vi "UI_(04A)_Set_Stop_State.vi"(3 "error in (no error)":errorcluster, 4 "Settings cluster in":T1={"Defaults"={"Default User"=0.0, "VISA Resource Name "=""}, "Recording and saving"={"Researcher name"="", "Name prefix"="", "Data post-processing"={"Filter type"=enum."Savitzky-Golay", "Length"=31, "Order"=3}, "Stop at"=0.0, "\"Stop at\" enabled"=FALSE, "Default save folder path"=path "", "Acquisition FPS"=enum."Max"}, "Geometry"={"Cage diameter, mm"=0, "Starting angle MIDFIELD"=0, "Starting angle BORDER"=0, "Radius, mm CENTER"=0, "Radius, mm MIDFIELD"=0, "N segments MIDFIELD"=0, "N segments BORDER"=0, "R-gap, mm"=0.0, "Bridge swap"=FALSE, "Bridge H. offset"=0.0, "Bridge V. offset"=0.0, "Twisted neck"=FALSE, "Alt. magn. orientation"=FALSE, "Sensor board size"=enum."Small"}, "IO parameters"={"IO general config."=0, "IO 1 configuration"=0, "IO 2 configuration"=0, "IO 3 configuration"=0, "IO 4 configuration"=0, "Activate ext. RS-232"=0, "IO inversion config."=0, "Sync capability"=1}, "Conditions presets array"=[{"Enabled"=FALSE, "Name"="", "Specifier(s)"=[], "Response"={"Response type"=enum."None", "TTL pulse length, ms"=0.0}}, {"Enabled"=FALSE, "Name"="", "Specifier(s)"=[], "Response"={"Response type"=enum."None", "TTL pulse length, ms"=0.0}}, {"Enabled"=FALSE, "Name"="", "Specifier(s)"=[], "Response"={"Response type"=enum."None", "TTL pulse length, ms"=0.0}}, {"Enabled"=FALSE, "Name"="", "Specifier(s)"=[], "Response"={"Response type"=enum."None", "TTL pulse length, ms"=0.0}}, {"Enabled"=FALSE, "Name"="", "Specifier(s)"=[], "Response"={"Response type"=enum."None", "TTL pulse length, ms"=0.0}}, {"Enabled"=FALSE, "Name"="", "Specifier(s)"=[], "Response"={"Response type"=enum."None", "TTL pulse length, ms"=0.0}}, {"Enabled"=FALSE, "Name"="", "Specifier(s)"=[], "Response"={"Response type"=enum."None", "TTL pulse length, ms"=0.0}}, {"Enabled"=FALSE, "Name"="", "Specifier(s)"=[], "Response"={"Response type"=enum."None", "TTL pulse length, ms"=0.0}}, {"Enabled"=FALSE, "Name"="", "Specifier(s)"=[], "Response"={"Response type"=enum."None", "TTL pulse length, ms"=0.0}}, {"Enabled"=FALSE, "Name"="", "Specifier(s)"=[], "Response"={"Response type"=enum."None", "TTL pulse length, ms"=0.0}}, {"Enabled"=FALSE, "Name"="", "Specifier(s)"=[], "Response"={"Response type"=enum."None", "TTL pulse length, ms"=0.0}}, {"Enabled"=FALSE, "Name"="", "Specifier(s)"=[], "Response"={"Response type"=enum."None", "TTL pulse length, ms"=0.0}}, {"Enabled"=FALSE, "Name"="", "Specifier(s)"=[], "Response"={"Response type"=enum."None", "TTL pulse length, ms"=0.0}}, {"Enabled"=FALSE, "Name"="", "Specifier(s)"=[], "Response"={"Response type"=enum."None", "TTL pulse length, ms"=0.0}}], "Calibration parameters"={"Timing calibration sw/hw"=1.0, "True FPS"=80.0, "True frame time, s"=80.0, "Disp. calibration info"=[]}, "Settings loaded OK"=FALSE} {"Calibration parameters"."True frame time, s" format="%.10g"; "Calibration parameters"."Disp. calibration info"."Speed, µl per ms" format="%.3g"; "Calibration parameters"."True FPS" format="%.10g"; "Calibration parameters"."Timing calibration sw/hw" format="%.10g"; "Conditions presets array"."Response"."TTL pulse length, ms" min=0.0 max=10000.0 step=10.0 format="%0.0g"; "Conditions presets array"."Specifier(s)"."Validity criteria(s)"."Validity value" min=0.0 step=0.1 format="%.2g"; "Conditions presets array"."Specifier(s)"."Value" step=1.0 format="%#.2g"; "Recording and saving"."Data post-processing"."Order" min=3 max=11 step=2; "Recording and saving"."Data post-processing"."Length" min=5 max=301 step=2; "Geometry"."Cage diameter, mm" scale=0.0..340.0}, 5 "All references in":T16) -> (0 "error out":errorcluster, 1 "Settings cluster out":T1={"Defaults"={"Default User"=0.0, "VISA Resource Name "=""}, "Recording and saving"={"Researcher name"="", "Name prefix"="", "Data post-processing"={"Filter type"=enum."Savitzky-Golay", "Length"=31, "Order"=3}, "Stop at"=0.0, "\"Stop at\" enabled"=FALSE, "Default save folder path"=path "", "Acquisition FPS"=enum."Max"}, "Geometry"={"Cage diameter, mm"=0, "Starting angle MIDFIELD"=0, "Starting angle BORDER"=0, "Radius, mm CENTER"=0, "Radius, mm MIDFIELD"=0, "N segments MIDFIELD"=0, "N segments BORDER"=0, "R-gap, mm"=0.0, "Bridge swap"=FALSE, "Bridge H. offset"=0.0, "Bridge V. offset"=0.0, "Twisted neck"=FALSE, "Alt. magn. orientation"=FALSE, "Sensor board size"=enum."Small"}, "IO parameters"={"IO general config."=0, "IO 1 configuration"=0, "IO 2 configuration"=0, "IO 3 configuration"=0, "IO 4 configuration"=0, "Activate ext. RS-232"=0, "IO inversion config."=0, "Sync capability"=1}, "Conditions presets array"=[{"Enabled"=FALSE, "Name"="", "Specifier(s)"=[], "Response"={"Response type"=enum."None", "TTL pulse length, ms"=0.0}}, {"Enabled"=FALSE, "Name"="", "Specifier(s)"=[], "Response"={"Response type"=enum."None", "TTL pulse length, ms"=0.0}}, {"Enabled"=FALSE, "Name"="", "Specifier(s)"=[], "Response"={"Response type"=enum."None", "TTL pulse length, ms"=0.0}}, {"Enabled"=FALSE, "Name"="", "Specifier(s)"=[], "Response"={"Response type"=enum."None", "TTL pulse length, ms"=0.0}}, {"Enabled"=FALSE, "Name"="", "Specifier(s)"=[], "Response"={"Response type"=enum."None", "TTL pulse length, ms"=0.0}}, {"Enabled"=FALSE, "Name"="", "Specifier(s)"=[], "Response"={"Response type"=enum."None", "TTL pulse length, ms"=0.0}}, {"Enabled"=FALSE, "Name"="", "Specifier(s)"=[], "Response"={"Response type"=enum."None", "TTL pulse length, ms"=0.0}}, {"Enabled"=FALSE, "Name"="", "Specifier(s)"=[], "Response"={"Response type"=enum."None", "TTL pulse length, ms"=0.0}}, {"Enabled"=FALSE, "Name"="", "Specifier(s)"=[], "Response"={"Response type"=enum."None", "TTL pulse length, ms"=0.0}}, {"Enabled"=FALSE, "Name"="", "Specifier(s)"=[], "Response"={"Response type"=enum."None", "TTL pulse length, ms"=0.0}}, {"Enabled"=FALSE, "Name"="", "Specifier(s)"=[], "Response"={"Response type"=enum."None", "TTL pulse length, ms"=0.0}}, {"Enabled"=FALSE, "Name"="", "Specifier(s)"=[], "Response"={"Response type"=enum."None", "TTL pulse length, ms"=0.0}}, {"Enabled"=FALSE, "Name"="", "Specifier(s)"=[], "Response"={"Response type"=enum."None", "TTL pulse length, ms"=0.0}}, {"Enabled"=FALSE, "Name"="", "Specifier(s)"=[], "Response"={"Response type"=enum."None", "TTL pulse length, ms"=0.0}}], "Calibration parameters"={"Timing calibration sw/hw"=1.0, "True FPS"=80.0, "True frame time, s"=80.0, "Disp. calibration info"=[]}, "Settings loaded OK"=FALSE} {"Calibration parameters"."True frame time, s" format="%.10g"; "Calibration parameters"."Disp. calibration info"."Speed, µl per ms" format="%.3g"; "Calibration parameters"."True FPS" format="%.10g"; "Calibration parameters"."Timing calibration sw/hw" format="%.10g"; "Conditions presets array"."Response"."TTL pulse length, ms" min=0.0 max=10000.0 step=10.0 format="%0.0g"; "Conditions presets array"."Specifier(s)"."Validity criteria(s)"."Validity value" min=0.0 step=0.1 format="%.2g"; "Conditions presets array"."Specifier(s)"."Value" step=1.0 format="%#.2g"; "Recording and saving"."Data post-processing"."Order" min=3 max=11 step=2; "Recording and saving"."Data post-processing"."Length" min=5 max=301 step=2; "Geometry"."Cage diameter, mm" scale=0.0..340.0}, 2 "All references out":T16)   [LabVIEW 2018, in "Tracker.lvlib"]
uses:
  Tracker.lvlib
  Controls/CTL_All_References.ctl
  Controls/CTL_Controls_References.ctl
  Controls/CTL_Indicators_References.ctl
  Controls/CTL_Panes_and_VIs_References.ctl
  Controls/CTL_Histogram_Properties.ctl
  <vilib>/Utility/miscctls.llb/LVRangeTypeDef.ctl
  Controls/CTL_Settings_cluster.ctl
  Controls/CTL_Filter_selector.ctl
  Controls/CTL_Acquisition_speed_selector.ctl
  Controls/CTL_Segmented_plot_parameters.ctl
  Controls/CTL_IO_params_cluster.ctl
  Controls/CTL_Conditions_Array.ctl
  Controls/CTL_Conditions_Cluster.ctl
  Controls/CTL_Condition_type.ctl
  Controls/CTL_Comparison_type.ctl
  Controls/CTL_Validity_check_criteria.ctl
  Controls/CTL_Condition_response_type.ctl
  Controls/CTL_Calibration_parameters.ctl
  Controls/CTL_Dispenser_calibration_info.ctl
  <vilib>/Utility/error.llb/Error Cluster From Error Code.vi
  <vilib>/ErrorRing/Error Ring.xnode
panel:
  in  "Histogram initialization cluster":T14={"X Scale.Range"={"Minimum"=0.0, "Maximum"=13.0, "Increment"=1.0, "Minor Increment"=1.0, "Start"=0.0}, "Caption.Text"="Zone preference (normalized)", "X Scale.Offset and Multiplier:Multiplier"=1.0, "X Scale.Offset and Multiplier:Offset"=0.0, "X Scale.Scale Fit"=2, "X Scale.Display Format:Precision"=0, "Y Scale.Mapping Mode"=0, "Zones preference empty initialized array"=[0, 0, 0, 0, 0, 0, 0, 0, 0, 0, 0, 0, 0, 0], "Plot.Fill/Point Color"=15790320}
  out "Panes references":T19
  out "Controls references params":string[][](array[string])
  out "Indicators references params":string[][](array[string])
  out "Indicators references":T18
  out "Controls references":T17
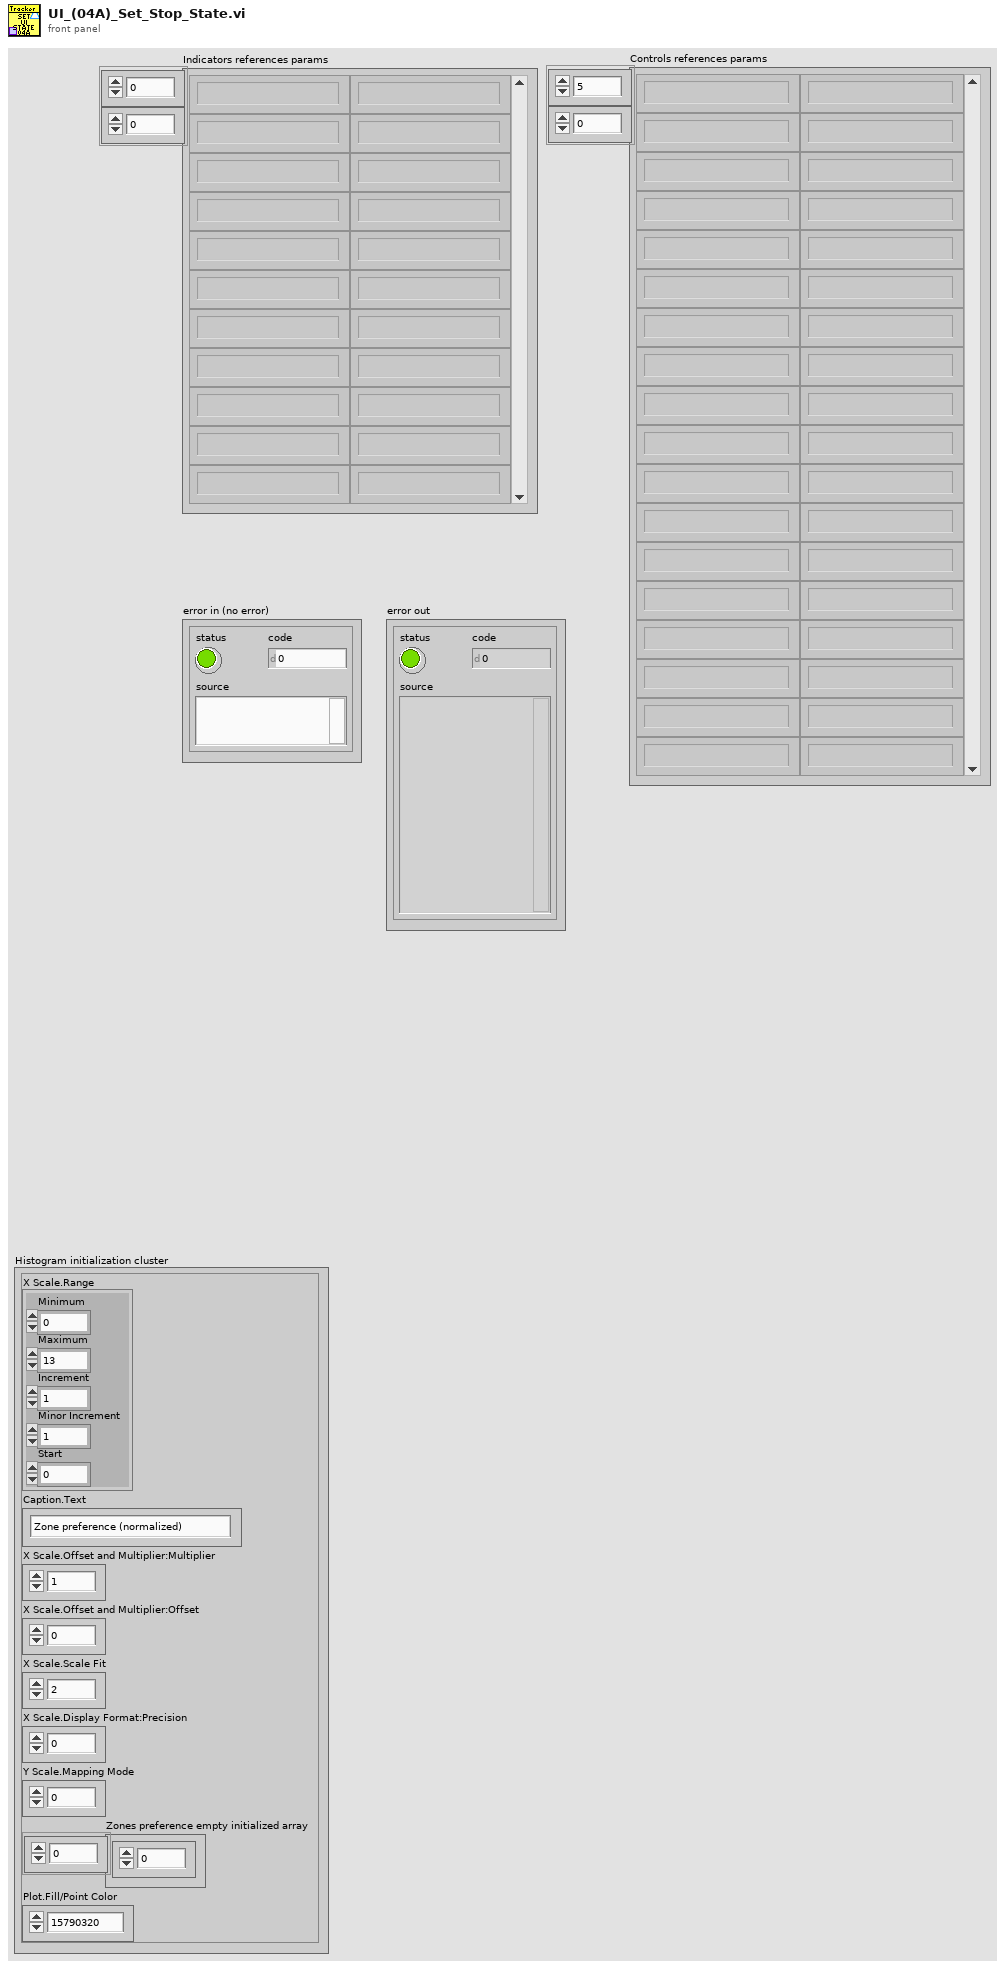
[diagram p1: front panel]
types:
  T1 = typedef "Tracker.lvlib/CTL_Settings_cluster.ctl" = cluster{"Defaults":cluster{"Default User":dbl, "VISA Resource Name ":string}, "Recording and saving":cluster{"Researcher name":string, "Name prefix":string, "Data post-processing":T2, "Stop at":dbl, "\"Stop at\" enabled":bool, "Default save folder path":path, "Acquisition FPS":T3}, "Geometry":T4, "IO parameters":T5, "Conditions presets array":T6, "Calibration parameters":T12, "Settings loaded OK":bool}
  T2 = typedef "Tracker.lvlib/CTL_Filter_selector.ctl" = cluster{"Filter type":enum16{"None", "Savitzky-Golay"}, "Length":i32, "Order":i32}
  T3 = typedef "Tracker.lvlib/CTL_Acquisition_speed_selector.ctl" = enum16{"Max", "Optimal", "Eco"}
  T4 = typedef "Tracker.lvlib/CTL_Segmented_plot_parameters.ctl" = cluster{"Cage diameter, mm":u16, "Starting angle MIDFIELD":i16, "Starting angle BORDER":i16, "Radius, mm CENTER":u16, "Radius, mm MIDFIELD":u16, "N segments MIDFIELD":u8, "N segments BORDER":u8, "R-gap, mm":sgl, "Bridge swap":bool, "Bridge H. offset":sgl, "Bridge V. offset":sgl, "Twisted neck":bool, "Alt. magn. orientation":bool, "Sensor board size":enum16{"Small", "Large"}}
  T5 = typedef "Tracker.lvlib/CTL_IO_params_cluster.ctl" = cluster{"IO general config.":u16, "IO 1 configuration":u16, "IO 2 configuration":u16, "IO 3 configuration":u16, "IO 4 configuration":u16, "Activate ext. RS-232":u16, "IO inversion config.":u16, "Sync capability":u8}
  T6 = typedef "Tracker.lvlib/CTL_Conditions_Array.ctl" = T7[]
  T7 = typedef "Tracker.lvlib/CTL_Conditions_Cluster.ctl" = cluster{"Enabled":bool, "Name":string, "Specifier(s)":cluster{"Specifier enabled":bool, "Condition type":T8, "Limit type":T9, "Value":dbl, "Validity criteria(s)":cluster{"V. check enabled":bool, "Criteria":T10, "Validity value":dbl}[]}[], "Response":cluster{"Response type":T11, "TTL pulse length, ms":dbl}}
  T8 = typedef "Tracker.lvlib/CTL_Condition_type.ctl" = enum16{"Not in use", "Speed", "Zone", "Angle to wall"}
  T9 = typedef "Tracker.lvlib/CTL_Comparison_type.ctl" = enum16{"Less", "Less or Equal", "Equal", "Greater or Equal", "Greater", "Not Equal"}
  T10 = typedef "Tracker.lvlib/CTL_Validity_check_criteria.ctl" = enum16{"Running bout (seconds)", "Running bout (meters)"}
  T11 = typedef "Tracker.lvlib/CTL_Condition_response_type.ctl" = enum16{"None", "TTL"}
  T12 = typedef "Tracker.lvlib/CTL_Calibration_parameters.ctl" = cluster{"Timing calibration sw/hw":dbl, "True FPS":dbl, "True frame time, s":dbl, "Disp. calibration info":T13}
  T13 = typedef "Tracker.lvlib/CTL_Dispenser_calibration_info.ctl" = cluster{"Channel":u8, "Speed, µl per ms":dbl}[]
  T14 = typedef "Tracker.lvlib/CTL_Histogram_Properties.ctl" = cluster{"X Scale.Range":T15, "Caption.Text":string, "X Scale.Offset and Multiplier:Multiplier":dbl, "X Scale.Offset and Multiplier:Offset":dbl, "X Scale.Scale Fit":u8, "X Scale.Display Format:Precision":u8, "Y Scale.Mapping Mode":u8, "Zones preference empty initialized array":i32[], "Plot.Fill/Point Color":u32}
  T15 = typedef "LVRangeTypeDef.ctl" = cluster{"Minimum":dbl, "Maximum":dbl, "Increment":dbl, "Minor Increment":dbl, "Start":dbl}
  T16 = typedef "Tracker.lvlib/CTL_All_References.ctl" = cluster{"Controls references":T17, "Indicators references":T18, "Service references":T19}
  T17 = typedef "Tracker.lvlib/CTL_Controls_References.ctl" = cluster{"Check HW connection":refnum<vi>, "Save settings":refnum<vi>, "Reset zones":refnum<vi>, "Reset stimuli":refnum<vi>, "Record/Stop":refnum<vi>, "Reset barplot":refnum<vi>, "Multiplyer of chart RX":refnum<vi>, "Show zones":refnum<vi>, "Show magnets":refnum<vi>, "Show heatmap":refnum<vi>, "Show full track":refnum<vi>, "Open File":refnum<vi>, "Play/Pause":refnum<vi>, "Trace, s":refnum<vi>, "Playback speed":refnum<vi>, "Timeline":refnum<vi>, "By Zone stim. setup":refnum<vi>, "Set/Rec and Analyse Tab":refnum<vi>, "Cage radial segmentation":refnum<vi>, "Set IO config":refnum<vi>, "Rainbow (time)":refnum<vi>, "Rainbow (speed)":refnum<vi>, "Add Reward":refnum<vi>, "Modify Reward":refnum<vi>, "Delete Reward":refnum<vi>}
  T18 = typedef "Tracker.lvlib/CTL_Indicators_References.ctl" = cluster{"HW info":refnum<vi>, "Port":refnum<vi>, "Ready":refnum<vi>, "IO status indicator":refnum<vi>, "Current Time":refnum<vi>, "Record timestamp":refnum<vi>, "Mouse speed":refnum<vi>, "Mouse speed, mm/s":refnum<vi>, "Running, perc. of time":refnum<vi>, "Histograms":refnum<vi>, "Cage size":refnum<vi>, "Reward":refnum<vi>}
  T19 = typedef "Tracker.lvlib/CTL_Panes_and_VIs_References.ctl" = cluster{"Pane":refnum<vi>, "This VI":refnum<vi>, "Menu":refnum<k9>}
  T20 = enum8{"Enabled", "Disabled", "Disabled and Grayed Out"}
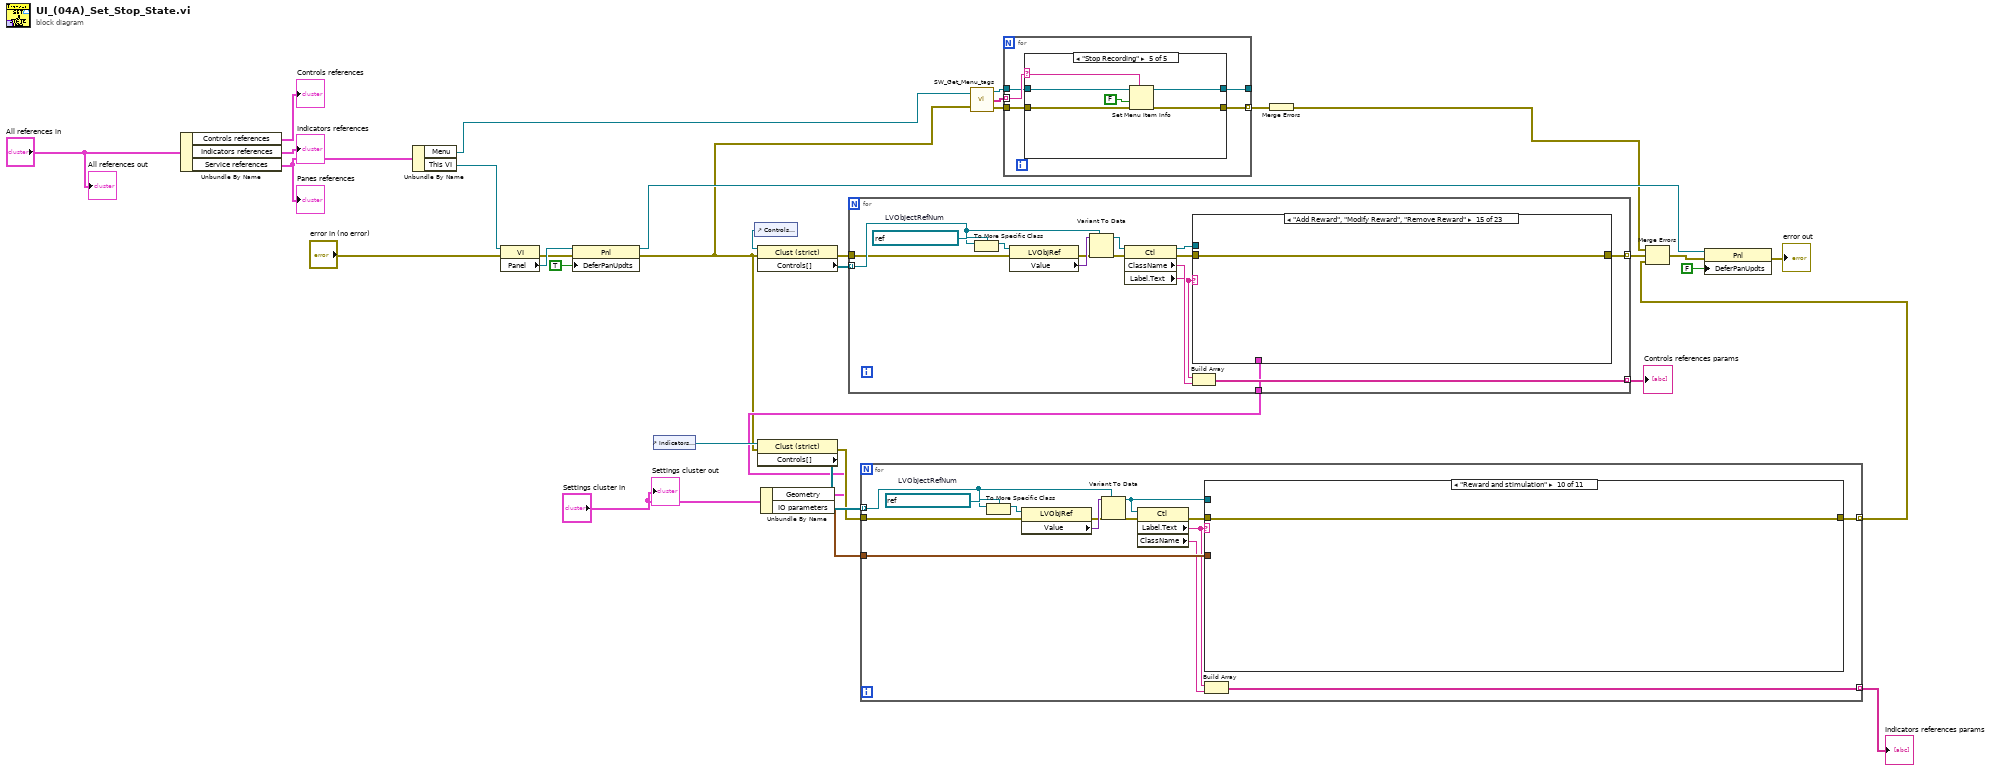
[diagram p0: block diagram]
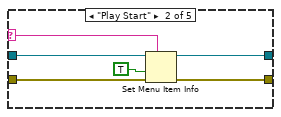
[diagram p3: hidden frame]
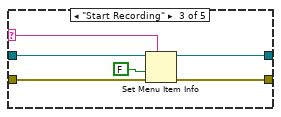
[diagram p4: hidden frame]
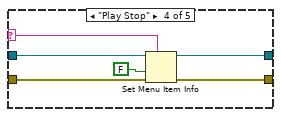
[diagram p5: hidden frame]
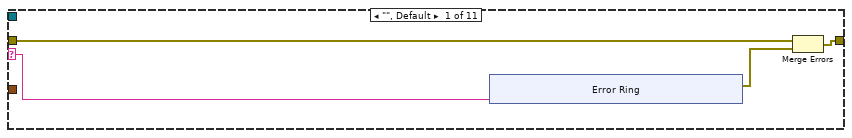
[diagram p6: hidden frame]
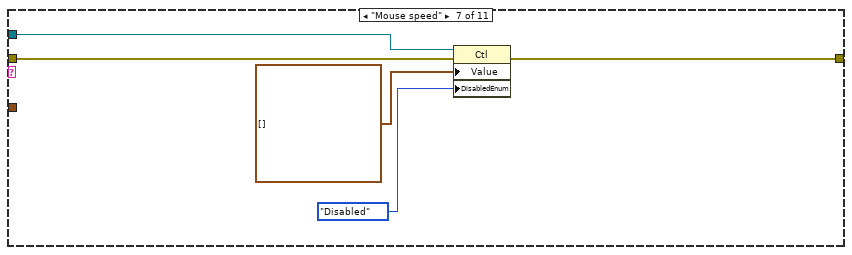
[diagram p12: hidden frame]
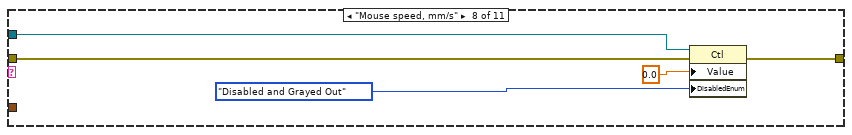
[diagram p13: hidden frame]
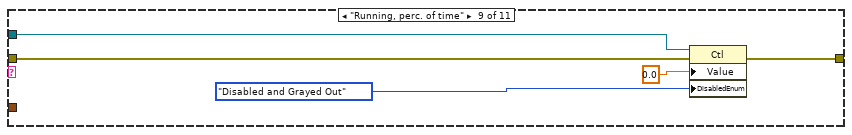
[diagram p14: hidden frame]
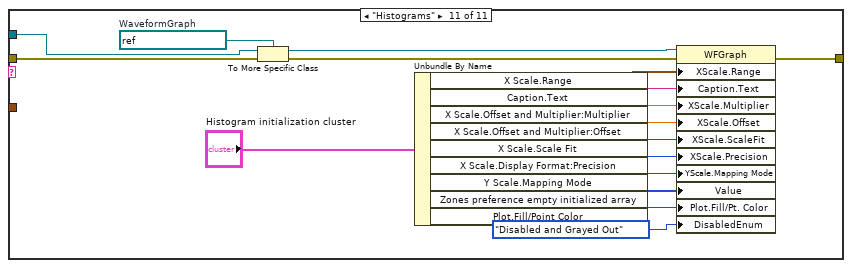
[diagram p15: hidden frame]
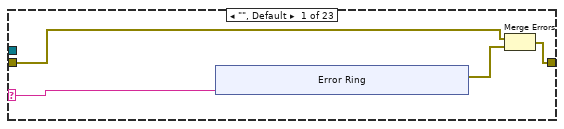
[diagram p16: hidden frame]
diagram:
  n1 = Unbundle By Name("All references in") -> ("Controls references"=→"Controls references":T17, "Indicators references"=→"Indicators references":T18, "Service references"=w24:T19)
  "Panes references" <- w24
  n2 = Unbundle By Name(w24) -> ("Menu"=w4:refnum<k9>, "This VI"=w21:refnum<vi>)
  n3 = property class="VI"(reference=w21, error in="error in (no error)") -> (error out=w15:errorcluster, "Panel"=w23:refnum<vi>)  [unwired: 1 out]
  n4 = property class="Pnl"(reference=w23, error in=w15, "DeferPanUpdts"=TRUE ("Defer Panel Updates")) -> (reference out=w16:refnum<vi>, error out=w3:errorcluster)
  n5 = control-ref of="Indicators references"() -> (w27:refnum<vi>)
  n6 = control-ref of="Controls references"() -> (w29:refnum<vi>)
  n7 = property class="Clust (strict)"(reference=w29, error in=w3) -> (error out=w20:errorcluster, "Controls[]"=w30:refnum<vi>[])  [unwired: 1 out]
  n8 = property class="Clust (strict)"(reference=w27, error in=w3) -> (error out=w19:errorcluster, "Controls[]"=w28:refnum<vi>[])  [unwired: 1 out]
  n9 = Unbundle By Name("Settings cluster in") -> ("Geometry"=w9:T4, "IO parameters"=w11:T5)
  n10 = for {
    tunnel: w30 -> [w45] mode=indexing
    tunnel: [w42] -> w25 mode=indexing
    tunnel: w20 -> [w41]
    tunnel: [w37] -> w13 mode=indexing
    tunnel: w9 -> [w34]
    w47 = refnum<vi> refnum  # LVObjectRefNum
    n11 = To More Specific Class(target class=w47, reference=w45) -> (specific class reference=w48:refnum<vi>)  [unwired: 1 in, 1 out]
    n12 = property class="LVObjRef"(reference=w48, error in=w41) -> (error out=w40:errorcluster, "Value"=w46:variant)  [unwired: 1 out]
    n13 = Variant To Data(error in=w40, type=w45, Variant=w46) -> (data=w44:refnum<vi>, error out=w39:errorcluster)
    n14 = property class="Ctl"(reference=w44, error in=w39) -> (reference out=w35:refnum<vi>, error out=w36:errorcluster, "ClassName"=w43:string, "Label.Text"=w38:string)
    n15 = case shown="\"Add Reward\", \"Modify Reward\", \"Remove Reward\"" w38 {
      selector: w38 -> [w49 _ _ _ _ _ _ _ _ _ _ _ _ _ _ _ _ _ _ _ _ _ _]
      tunnel: [w51 w60 w61 w62 w63 w64 w65 w66 w69 w77 w85 w91 w92 w93 w100 w103 w111 w117 w125 w128 w136 w143 w149] -> w37
      tunnel: w36 -> [w52 w60 w61 w62 w63 w64 w65 w66 w71 w79 w87 w91 w92 w94 w100 w105 w113 w119 w125 w130 w138 w145 w149]
      tunnel: w35 -> [_ _ _ _ _ _ _ _ w74 w82 w90 _ _ w95 _ w108 w116 w118 _ w133 w141 w148 _]
      tunnel: w34 -> [_ _ _ _ _ _ _ _ _ _ _ _ _ _ _ _ _ _ _ _ _ _ _]
      frame "", Default {
        n16 = xnode "Error Ring"("parameter 0"=w49) -> ("error out"=w50:errorcluster)
        n17 = Merge Errors(w52, w50) -> (w51:errorcluster)
      }
      frame "Cage radial segmentation" {
      }
      frame "Set/Rec and Analyse Tab" {
      }
      frame "Check HW connection" {
      }
      frame "Save settings" {
      }
      frame "Set IO config" {
      }
      frame "Reset zones" {
      }
      frame "Reset stimuli" {
      }
      frame "Record/Stop" {
        w73 = refnum<vi> refnum  # Boolean
        n18 = To More Specific Class(target class=w73, reference=w74, error in=w71) -> (specific class reference=w72:refnum<vi>, error out=w70:errorcluster)
        n19 = property class="Bool"(reference=w72, error in=w70, "Value"=FALSE, "DisabledEnum"=T20."Disabled and Grayed Out" ("Disabled")) -> (error out=w69:errorcluster)  [unwired: 1 out]
      }
      frame "Reset barplot" {
        w81 = refnum<vi> refnum  # Boolean
        n20 = To More Specific Class(target class=w81, reference=w82, error in=w79) -> (specific class reference=w80:refnum<vi>, error out=w78:errorcluster)
        n21 = property class="Bool"(reference=w80, error in=w78, "Value"=FALSE, "DisabledEnum"=T20."Disabled and Grayed Out" ("Disabled")) -> (error out=w77:errorcluster)  [unwired: 1 out]
      }
      frame "Multiplyer of chart RX" {
        w89 = refnum<vi> refnum  # Slide
        n22 = To More Specific Class(target class=w89, reference=w90, error in=w87) -> (specific class reference=w88:refnum<vi>, error out=w86:errorcluster)
        n23 = property class="Slide"(reference=w88, error in=w86, "Value"=u8 1, "DisabledEnum"=T20."Disabled and Grayed Out" ("Disabled")) -> (error out=w85:errorcluster)  [unwired: 1 out]
      }
      frame "Show zones" {
      }
      frame "Show magnets" {
      }
      frame "Rainbow (speed)", "Rainbow (time)" {
        w96 = refnum<vi> refnum  # Boolean
        n24 = To More Specific Class(target class=w96, reference=w95, error in=w94) -> (specific class reference=w99:refnum<vi>, error out=w98:errorcluster)
        n25 = property class="Bool"(reference=w99, error in=w98, "DisabledEnum"=T20."Disabled and Grayed Out" ("Disabled")) -> (error out=w93:errorcluster)  [unwired: 1 out]
      }
      frame "Add Reward", "Modify Reward", "Remove Reward" {
      }
      frame "Show heatmap" {
        w107 = refnum<vi> refnum  # Boolean
        n26 = To More Specific Class(target class=w107, reference=w108, error in=w105) -> (specific class reference=w106:refnum<vi>, error out=w104:errorcluster)
        n27 = property class="Bool"(reference=w106, error in=w104, "Value"=FALSE, "DisabledEnum"=T20."Disabled and Grayed Out" ("Disabled")) -> (error out=w103:errorcluster)  [unwired: 1 out]
      }
      frame "Show full track" {
        w115 = refnum<vi> refnum  # Boolean
        n28 = To More Specific Class(target class=w115, reference=w116, error in=w113) -> (specific class reference=w114:refnum<vi>, error out=w112:errorcluster)
        n29 = property class="Bool"(reference=w114, error in=w112, "Value"=FALSE, "DisabledEnum"=T20."Disabled and Grayed Out" ("Disabled")) -> (error out=w111:errorcluster)  [unwired: 1 out]
      }
      frame "Open File" {
        w120 = refnum<vi> refnum  # Boolean
        n30 = To More Specific Class(target class=w120, reference=w118, error in=w119) -> (specific class reference=w124:refnum<vi>, error out=w123:errorcluster)
        n31 = property class="Bool"(reference=w124, error in=w123, "Value"=FALSE, "DisabledEnum"=T20."Enabled" ("Disabled")) -> (error out=w117:errorcluster)  [unwired: 1 out]
      }
      frame "Play/Pause" {
      }
      frame "Trace, s" {
        w132 = refnum<vi> refnum  # Slide
        n32 = To More Specific Class(target class=w132, reference=w133, error in=w130) -> (specific class reference=w131:refnum<vi>, error out=w129:errorcluster)
        n33 = property class="Slide"(reference=w131, error in=w129, "Value"=u8 5, "DisabledEnum"=T20."Disabled and Grayed Out" ("Disabled")) -> (error out=w128:errorcluster)  [unwired: 1 out]
      }
      frame "Playback speed" {
        w140 = refnum<vi> refnum  # Ring
        n34 = To More Specific Class(target class=w140, reference=w141, error in=w138) -> (specific class reference=w139:refnum<vi>, error out=w137:errorcluster)
        n35 = property class="Ring"(reference=w139, error in=w137, "Value"=u8 3, "DisabledEnum"=T20."Disabled and Grayed Out" ("Disabled")) -> (error out=w136:errorcluster)  [unwired: 1 out]
      }
      frame "Timeline" {
        w147 = refnum<vi> refnum  # Slide
        n36 = To More Specific Class(target class=w147, reference=w148, error in=w145) -> (specific class reference=w146:refnum<vi>, error out=w144:errorcluster)
        n37 = property class="Slide"(reference=w146, error in=w144, "DisabledEnum"=T20."Disabled and Grayed Out" ("Disabled")) -> (error out=w143:errorcluster)  [unwired: 1 out]
      }
      frame "By Zone stim. setup" {
      }
    }
    n38 = Build Array(w38, w43) -> (w42:string[])
  }
  "Controls references params" <- w25
  n39 = for {
    tunnel: w28 -> [w160] mode=indexing
    tunnel: [w150] -> w26 mode=indexing
    tunnel: w19 -> [w158]
    tunnel: [w154] -> w1 mode=indexing
    tunnel: w11 -> [w153]
    w162 = refnum<vi> refnum  # LVObjectRefNum
    n40 = To More Specific Class(target class=w162, reference=w160) -> (specific class reference=w163:refnum<vi>)  [unwired: 1 in, 1 out]
    n41 = property class="LVObjRef"(reference=w163, error in=w158) -> (error out=w157:errorcluster, "Value"=w161:variant)  [unwired: 1 out]
    n42 = Variant To Data(error in=w157, type=w160, Variant=w161) -> (data=w159:refnum<vi>, error out=w156:errorcluster)
    n43 = property class="Ctl"(reference=w159, error in=w156) -> (error out=w155:errorcluster, "Label.Text"=w152:string, "ClassName"=w151:string)  [unwired: 1 out]
    n44 = case shown="\"Reward and stimulation\"" w152 {
      selector: w152 -> [w164 _ _ _ _ _ _ _ _ _ _]
      tunnel: w159 -> [_ _ _ _ _ _ w184 w189 w194 _ w212]
      tunnel: w155 -> [w167 w175 w176 w177 w178 w179 w183 w188 w193 w195 w198]
      tunnel: [w166 w175 w176 w177 w178 w179 w182 w187 w192 w195 w211] -> w154
      tunnel: w153 -> [_ _ _ _ _ _ _ _ _ _ _]
      frame "", Default {
        n45 = xnode "Error Ring"("parameter 0"=w164) -> ("error out"=w165:errorcluster)
        n46 = Merge Errors(w167, w165) -> (w166:errorcluster)
      }
      frame "Cage size", "HW info", "Port" {
      }
      frame "Ready" {
      }
      frame "IO status indicator" {
      }
      frame "Current Time" {
      }
      frame "Since track start" {
      }
      frame "Mouse speed" {
        n47 = property class="Ctl"(reference=w184, error in=w183, "Value"=waveform(dbl)[] [] ("History Data"), "DisabledEnum"=T20."Disabled" ("Disabled")) -> (error out=w182:errorcluster)  [unwired: 1 out]
      }
      frame "Mouse speed, mm/s" {
        n48 = property class="Ctl"(reference=w189, error in=w188, "Value"=0.0, "DisabledEnum"=T20."Disabled and Grayed Out" ("Disabled")) -> (error out=w187:errorcluster)  [unwired: 1 out]
      }
      frame "Running, perc. of time" {
        n49 = property class="Ctl"(reference=w194, error in=w193, "Value"=0.0, "DisabledEnum"=T20."Disabled and Grayed Out" ("Disabled")) -> (error out=w192:errorcluster)  [unwired: 1 out]
      }
      frame "Reward and stimulation" {
      }
      frame "Histograms" {
        w209 = refnum<vi> refnum  # WaveformGraph
        n50 = To More Specific Class(target class=w209, reference=w212, error in=w198) -> (specific class reference=w210:refnum<vi>, error out=w197:errorcluster)
        n51 = Unbundle By Name("Histogram initialization cluster") -> ("X Scale.Range"=w207:T15, "Caption.Text"=w206:string, "X Scale.Offset and Multiplier:Multiplier"=w205:dbl, "X Scale.Offset and Multiplier:Offset"=w204:dbl, "X Scale.Scale Fit"=w203:u8, "X Scale.Display Format:Precision"=w202:u8, "Y Scale.Mapping Mode"=w201:u8, "Zones preference empty initialized array"=w200:i32[], "Plot.Fill/Point Color"=w199:u32)
        n52 = property class="WFGraph"(reference=w210, error in=w197, "XScale.Range"=w207, "Caption.Text"=w206, "XScale.Multiplier"=w205, "XScale.Offset"=w204, "XScale.ScaleFit"=w203, "XScale.Precision"=w202, "YScale.Mapping Mode"=w201, "Value"=w200, "Plot.Fill/Pt. Color"=w199, "DisabledEnum"=T20."Disabled and Grayed Out" ("Disabled")) -> (error out=w211:errorcluster)  [unwired: 1 out]
      }
    }
    n53 = Build Array(w152, w151) -> (w150:string[])
  }
  "Indicators references params" <- w26
  n54 = call "SW_Get_Menu_tags.vi"("Menu ref in"=w4, "error in (no error)"=w3) -> ("Menu ref out"=w6:refnum<k9>, "(Sub)menu tags"=w8:string[], "error out"=w7:errorcluster)
  n55 = for {
    tunnel: w8 -> [w217] mode=indexing
    tunnel: w7 -> [w216]
    tunnel: [w215] -> w5 mode=indexing
    tunnel: [w214] -> _
    tunnel: w6 -> [w213]
    n56 = case shown="\"Stop Recording\"" w217 {
      selector: w217 -> [_ w225 w231 w237 w243]
      tunnel: w216 -> [w219 w223 w229 w235 w241]
      tunnel: [w219 w222 w228 w234 w240] -> w215
      tunnel: [w218 w221 w227 w233 w239] -> w214
      tunnel: w213 -> [w218 w220 w226 w232 w238]
      frame "", Default {
      }
      frame "Play Start" {
        n57 = Set Menu Item Info(7:w225, 8:w223, 9:TRUE ("enabled"), 11:w220) -> (0:w222:errorcluster, 3:w221:refnum<k9>)  [unwired: 3 in]
      }
      frame "Start Recording" {
        n58 = Set Menu Item Info(7:w231, 8:w229, 9:FALSE ("enabled"), 11:w226) -> (0:w228:errorcluster, 3:w227:refnum<k9>)  [unwired: 3 in]
      }
      frame "Play Stop" {
        n59 = Set Menu Item Info(7:w237, 8:w235, 9:FALSE ("enabled"), 11:w232) -> (0:w234:errorcluster, 3:w233:refnum<k9>)  [unwired: 3 in]
      }
      frame "Stop Recording" {
        n60 = Set Menu Item Info(7:w243, 8:w241, 9:FALSE ("enabled"), 11:w238) -> (0:w240:errorcluster, 3:w239:refnum<k9>)  [unwired: 3 in]
      }
    }
  }
  n61 = Merge Errors(w5) -> (w2:errorcluster)
  n62 = Merge Errors(w2, w13, w1) -> (w18:errorcluster)
  n63 = property class="Pnl"(reference=w16, error in=w18, "DeferPanUpdts"=FALSE ("Defer Panel Updates")) -> (error out=→"error out":errorcluster)  [unwired: 1 out]
  "All references out" <- "All references in"
  "Settings cluster out" <- "Settings cluster in"
